vi "Access Data.vi"(8 "error in (no error)":errorcluster, 11 "Data to Access":refnum<class "Data.lvclass">) -> (0 "error out":errorcluster, 2 "Found?":bool, 3 "Data out":refnum<class "Data.lvclass">)   [LabVIEW 2020, in "Data Repository.lvlib"]
doc: "Access Data by Data alias and return the data if found."
uses:
  Data Repository.lvlib
  PPL/HDH.Data.Generic.lvlibp/Data.lvclass
  PPL/HDH.Data.Generic.lvlibp/Synchronization/Notifier/Notifier.lvclass
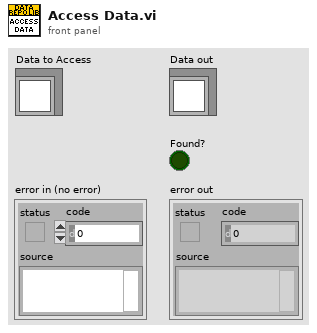
[diagram p1: front panel]
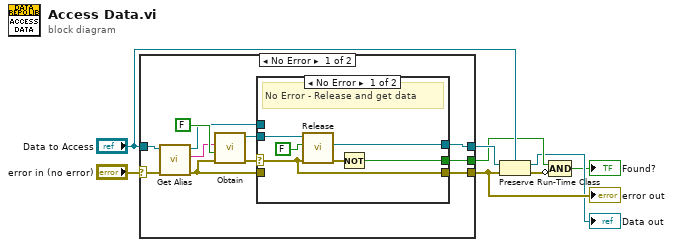
[diagram p0: block diagram]
diagram:
  n1 = case shown="No Error" "error in (no error)" {
    selector: "error in (no error)" -> [w16 w28]
    tunnel: "Data to Access" -> [w18 w29]
    tunnel: [w13 w29] -> w7
    tunnel: [w11 w28] -> w3
    tunnel: [w10 _] -> w5
    frame No Error {
      n2 = call-dynamic "Get Alias.vi"("error in (no error)"=w16, "Data in"=w18) -> ("error out"=w9:errorcluster, "Alias"=w17:string, "Data out"=w12:refnum<class "Data.lvclass">)  [unwired: 7 in]
      n3 = call "Obtain.vi"("error in (no error)"=w9, "create if not found? (T)"=FALSE, "Name (\"\")"=w17) -> ("error out"=w15:errorcluster, "Notifier out"=w14:refnum<class "Notifier.lvclass">)  [unwired: 6 in, 1 out]
      n4 = case shown="No Error" w15 {
        selector: w15 -> [w23 _]
        tunnel: w14 -> [w25 _]
        tunnel: [w24 w27] -> w13
        tunnel: w12 -> [_ w27]
        tunnel: [w23 w26] -> w11
        tunnel: [w20 _] -> w10
        tunnel: w9 -> [_ w26]
        frame No Error {
          # "No Error - Release and get data"
          n5 = call "Release.vi"("error in (no error)"=w23, "Force destroy? (F)"=FALSE ("Ignore previous (F)"), "Notifier in"=w25) -> ("error out"=w22:errorcluster, "Last Data Notification"=w24:refnum<class "Data.lvclass">)  [unwired: 6 in, 1 out]
          n6 = Not(x=w22) -> (.not. x?=w20:bool)
        }
        frame Error {
          # "Error - Notifier not found"
        }
      }
    }
    frame Error {
    }
  }
  "error out" <- w3
  n7 = Preserve Run-Time Class(object in=w7, error in=w3, 2:"Data to Access") -> (object out=→"Data out":refnum<class "Data.lvclass">, error out=w4:errorcluster)
  n8 = Compound Arithmetic op=AND(w5, invert w4) -> (→"Found?":bool)
